vi "DN4_AO_OneBufferedWrite.vi"(8 "error in (no error)":errorcluster, 9 "data in(DDT)":dynamicdata(waveform), 11 "Task ID":u32) -> (0 "error out":errorcluster, 3 "Task out ID":u32)   [LabVIEW 2009]
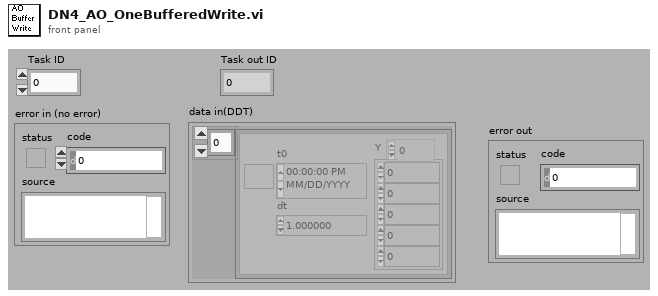
[diagram p1: front panel]
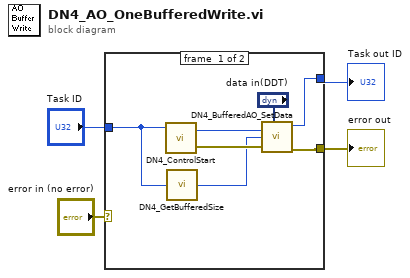
[diagram p0: block diagram]
diagram:
  n1 = case shown="No Error" "error in (no error)" {
    selector: "error in (no error)" -> [_ w12]
    tunnel: [w6 w13] -> w2
    tunnel: "Task ID" -> [w10 w13]
    tunnel: [w5 w12] -> w1
    frame #0 {
      n2 = call <userlib>:"DN4_ControlStart.vi"("Task ID"=w10) -> ("error out"=w9:errorcluster, "Task ID"=w8:u32)  [unwired: 1 in, 1 out]
      n3 = call <userlib>:"DN4_GetBufferedSize.vi"("Task ID"=w10) -> ("return type"=w7:i32)
      n4 = call <userlib>:"DN4_BufferedAO_SetData.vi"("data in(DDT)"="data in(DDT)", "error in (no error)"=w9, "count"=w7, "Task ID"=w8) -> ("error out"=w5:errorcluster, "Task ID"=w6:u32)  [unwired: 1 in, 5 out]
    }
    frame #1 {
    }
  }
  "error out" <- w1
  "Task out ID" <- w2
